vi "Pause Process.vi"(8 "error in (no error)":errorcluster, 11 "Process Model in":refnum<class "Process Model.lvclass">) -> (0 "error out":errorcluster, 3 "Process Model out":refnum<class "Process Model.lvclass">)   [LabVIEW 2017, in "Car Wash.lvlib" / "Process Model.lvlib" / "Process Model.lvclass"]
uses:
  Process Model.lvclass
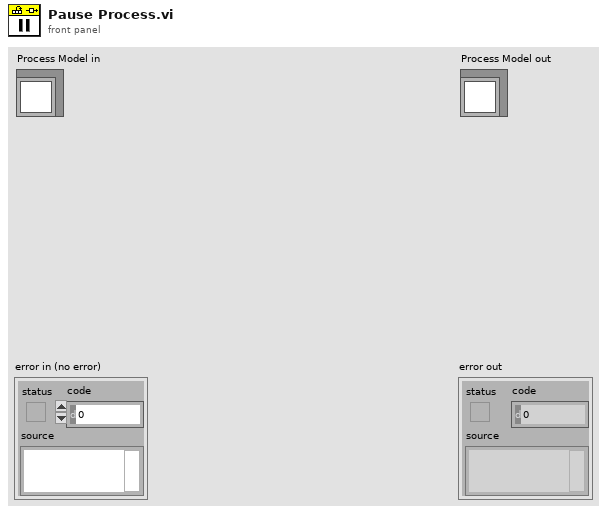
[diagram p1: front panel]
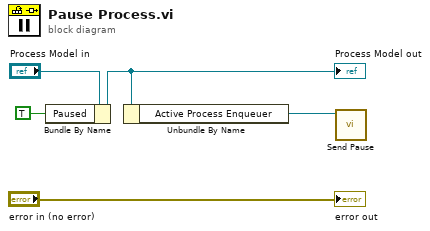
[diagram p0: block diagram]
diagram:
  n1 = Bundle By Name(cluster="Process Model in", "Paused"=TRUE) -> (w2:refnum<class "Process Model.lvclass">)
  "Process Model out" <- w2
  n2 = Unbundle By Name(w2) -> ("Active Process Enqueuer"=w1:refnum<class "Message Enqueuer.lvclass">)
  n3 = call "Send Pause.vi"("Message Enqueuer"=w1) -> ()  [unwired: 9 in, 2 out]
  "error out" <- "error in (no error)"
